vi "Read Entire File.vi"(5 "convert eoln (F)":bool, 8 "error in":errorcluster, 11 "path":path) -> (0 "error out":errorcluster, 2 "data":string, 3 "duplicate path":path, 4 "size":i32)   [LabVIEW 2015, in "TLB` Template.lvlib" / "Tools_String.lvlib"]
doc: "TLB Prime - Application Template 1.3.0.24\nNorm Kirchner, NI Systems Engineering - NI\nCopyright (c) 2014, NI"
uses:
  Tools_String.lvlib
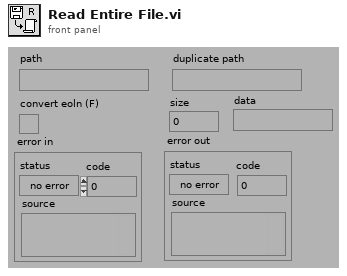
[diagram p1: front panel]
types:
  T1 = enum16{"read/write", "read-only", "write-only", "write-only (truncate)"}
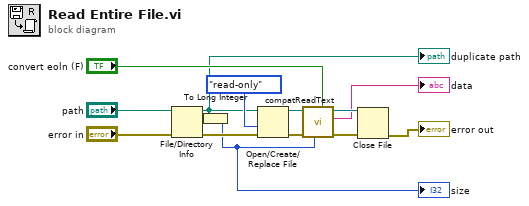
[diagram p0: block diagram]
diagram:
  n1 = File/Directory Info(path="path", error in="error in") -> (path out=w5:path, size=w1:i64, error out=w13:errorcluster)  [unwired: 4 out]
  "duplicate path" <- w5
  n2 = To Long Integer(number=w1) -> (32bit integer=w9:i32)
  "size" <- w9
  n3 = Open/Create/Replace File(file path (use dialog)=w5, error in=w13, access (0:read/write)=T1."read-only" ("open mode (0)")) -> (refnum out=w11:refnum<file>, error out=w10:errorcluster)  [unwired: 4 out]
  n4 = call <vilib>:"compatReadText.vi"("convert eol (F)"="convert eoln (F)", "count"=w9, "error in"=w10, "refnum"=w11) -> ("error out"=w7:errorcluster, "data"=→"data":string, "dup refnum"=w8:refnum<file>)  [unwired: 1 in, 4 out]
  n5 = Close File(refnum=w8, error in=w7) -> (error out=→"error out":errorcluster)  [unwired: 1 out]
